vi "frog analysis.vi"(3 "error in (no error)":errorcluster, 5 "FROG in":refnum<class "FROG.lvclass">) -> (0 "error out":errorcluster, 2 "FROG out":refnum<class "FROG.lvclass">)   [LabVIEW 2020, in "FROG.lvclass"]
uses:
  FROG.lvclass
  FROG.lvclass/FROG.ctl
  Point Grey Camera/GUIcompressionCluster.ctl
  shared/OnOffTypeDef.ctl
  shared/CompressAndUpdate(Poly)/CompressAndUpdate(NumericArray).vi
  shared/CompressAndUpdate(Poly)/CompressAndUpdate(IMAQ Image).vi
  shared/CompressAndUpdate(Poly)/CompressAndUpdate(Numeric).vi
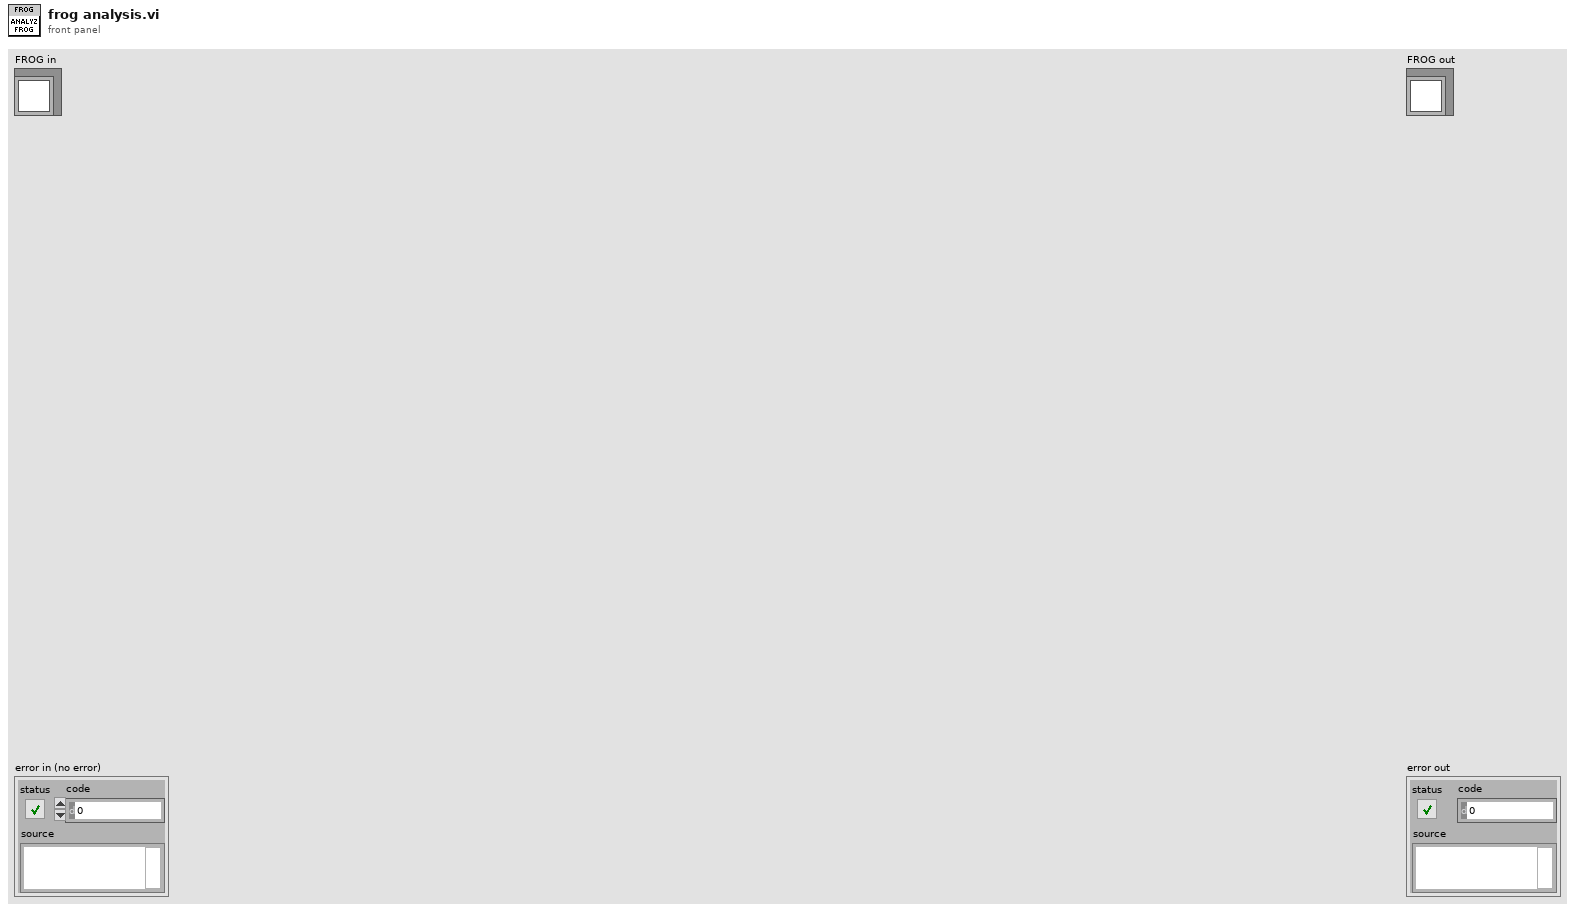
[diagram p1: front panel]
types:
  T1 = typedef "IMAQ Image.ctl" = refnum<image>
  T2 = typedef "GUIcompressionCluster.ctl" = cluster{"GUI8bit":T3, "GUICompression":T3, "CompressionQuality":i32}
  T3 = typedef "OnOffTypeDef.ctl" = enum16{"off", "on"}
  T4 = cluster{"waveout":dbl[], "specOut":dbl[], dbl[], "timeout":dbl[], "field":dbl[], dbl[]}
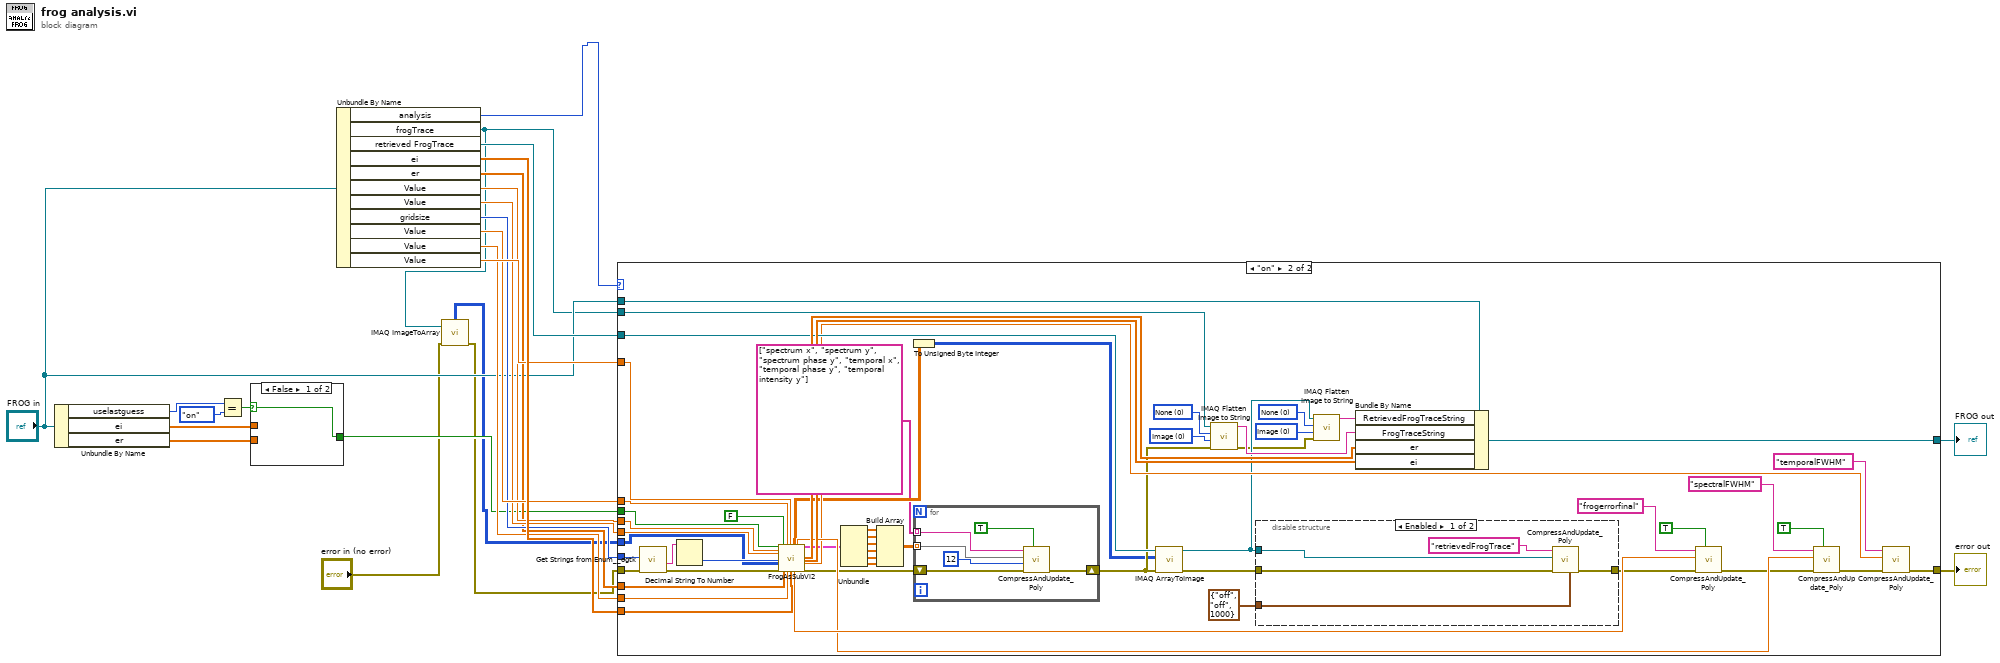
[diagram p0: block diagram]
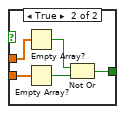
[diagram p2: hidden frame]
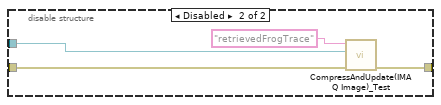
[diagram p4: hidden frame]
diagram:
  n1 = Unbundle By Name ("pressure read")("FROG in") -> ("uselastguess"=w10:enum16{"off", "on"}, "ei"=w9:dbl[], "er"=w8:dbl[])
  n2 = Equal?(x=w10, y=enum16{"off", "on"}."on" ("uselastguess")) -> (x = y?=w11:bool)
  n3 = case shown="False" w11 {
    selector: w11 -> [w24 _]
    tunnel: w9 -> [_ w25]
    tunnel: w8 -> [_ w29]
    tunnel: [w24 w26] -> w7
    frame False {
    }
    frame True {
      n4 = Empty Array?(array=w25) -> (empty?=w27:bool)
      n5 = Empty Array?(array=w29) -> (empty?=w28:bool)
      n6 = Not Or(1:w28, 2:w27) -> (0:w26:bool)
    }
  }
  n7 = Unbundle By Name ("pressure read")("FROG in") -> ("analysis"=w5:enum16{"off", "on"}, "frogTrace"=w4:T1, "retrieved FrogTrace"=w14:T1, "ei"=w21:dbl[], "er"=w13:dbl[], "Value"=w15:dbl, "Value"=w16:dbl, "gridsize"=w17:enum16{"64", "128", "256", "512"}, "Value"=w19:dbl, "Value"=w18:dbl, "Value"=w20:dbl)
  n8 = call "IMAQ ImageToArray"("error in (no error)"="error in (no error)", "Image"=w4) -> ("error out"=w1:errorcluster, "Image Pixels (U8)"=w3:u8[][])  [unwired: 2 in, 3 out]
  n9 = case shown="\"on\"" w5 {
    tunnel: "FROG in" -> [w31 w87]
    tunnel: [w31 w86] -> w22
    tunnel: w7 -> [_ w85]
    tunnel: w15 -> [_ w84]
    tunnel: w16 -> [_ w83]
    tunnel: w17 -> [_ w80]
    tunnel: w13 -> [_ w76]
    tunnel: w21 -> [_ w75]
    tunnel: w14 -> [_ w73]
    tunnel: [w30 w61] -> w23
    tunnel: w1 -> [w30 w51]
    tunnel: w19 -> [_ w49]
    tunnel: w20 -> [_ w48]
    tunnel: w18 -> [_ w47]
    tunnel: w4 -> [_ w42]
    tunnel: w3 -> [_ w34]
    frame "off", Default {
    }
    frame "on" {
      w39 = 0 items=["Image", "Image and Vision Info", "Reference to Image"] ("Type of Flatten (Image and Vision Info)")
      w38 = 0 items=["None", "JPEG", "PACKED BINARY"] ("Compression (None)")
      w43 = 0 items=["Image", "Image and Vision Info", "Reference to Image"] ("Type of Flatten (Image and Vision Info)")
      w44 = 0 items=["None", "JPEG", "PACKED BINARY"] ("Compression (None)")
      n10 = call <userlib>:"Get Strings from Enum__ogtk.vi"("error in (no error)"=w51, "Enum"=w80) -> ("error out"=w77:errorcluster, "String Value"=w79:string)  [unwired: 6 in, 2 out]
      n11 = Decimal String To Number(string=w79) -> (number=w78:i32)  [unwired: 2 in, 1 out]
      n12 = call "FrogAsSubVi2.vi"("use last retrieval as guess"=w85, "max time/retrieval [ms]"=w84, "set Frog error"=w83, "Grid size"=w78, "8-bit pixmap"=w34, "error in (no error)"=w77, "Stop"=FALSE, "er in"=w76, "delt"=w49, "dellam"=w47, "lam0"=w48, "ei in"=w75) -> ("retrieved Frog trace"=w60:dbl[][], "Best Frog Error"=w70:dbl, "spectral FWHM"=w67:dbl, "Temporal and Spatial Arrays"=w50:T4, "er"=w82:dbl[], "ei"=w81:dbl[], "temporal FWHM"=w65:dbl, "error out"=w46:errorcluster)  [unwired: 8 in]
      n13 = Unbundle(w50) -> ("waveout"=w59:dbl[], "specOut"=w58:dbl[], w57:dbl[], "timeout"=w56:dbl[], "field"=w55:dbl[], w54:dbl[])
      n14 = Build Array(w59, w58, w57, w56, w55, w54) -> (w53:dbl[][])
      n15 = To Unsigned Byte Integer(number=w60) -> (unsigned 8bit integer=w33:u8[][])
      n16 = for {
        tunnel: w53 -> [w101] mode=indexing
        tunnel: string[] ["spectrum x", "spectrum y", "spectrum phase y", "temporal x", "temporal phase y", "temporal intensity y"] -> [w102] mode=indexing
        shift-right: [w97] -> w41
        shift-left: w46 -> [w98]
        n17 = call-poly "CompressAndUpdate_Poly.vi"("force CVT update (false)"=TRUE, "error in"=w98, "precision (6)"=i16 12, "Numeric Array"=w101, "command or variable name"=w102) -> ("error out"=w97:errorcluster)  [unwired: 6 in]
      }
      n18 = call "IMAQ ArrayToImage"("error in (no error)"=w41, "Image Pixels (U8)"=w33, "Image"=w73) -> ("error out"=w64:errorcluster, "Image Out"=w37:T1)  [unwired: 7 in]
      n19 = call "IMAQ Flatten Image to String"("error in (no error)"=w41, "Type of Flatten (Image and Vision Info)"=w43, "Compression (None)"=w44, "Image"=w42) -> ("error out"=w36:errorcluster, "Data String"=w40:string)  [unwired: 6 in]
      n20 = disable-structure shown="Enabled" {
        disable-tunnel: w64 -> [w91 w96]
        disable-tunnel: [w90 w95] -> w45
        disable-tunnel: w37 -> [w89 w94]
        disable-tunnel: T2 {"GUI8bit"=enum."off", "GUICompression"=enum."off", "CompressionQuality"=1000} ("GUICompression") -> [w88 _]
        frame Enabled {
          n21 = call-poly "CompressAndUpdate_Poly.vi"("GUICompression"=w88, "error in"=w91, "IMAQ Image"=w89, "command or variable name"="retrievedFrogTrace") -> ("error out"=w90:errorcluster)  [unwired: 7 in]
        }
        frame Disabled {
          n22 = call "CompressAndUpdate(IMAQ Image)_Test.vi"("error in"=w96, "IMAQ Image"=w94, "command or variable name"="retrievedFrogTrace") -> ("error out"=w95:errorcluster)  [unwired: 8 in]
        }
      }
      n23 = call "IMAQ Flatten Image to String"("error in (no error)"=w36, "Type of Flatten (Image and Vision Info)"=w39, "Compression (None)"=w38, "Image"=w37) -> ("Data String"=w35:string)  [unwired: 6 in, 1 out]
      n24 = Bundle By Name(cluster=w87, "RetrievedFrogTraceString"=w35, "FrogTraceString"=w40, "er"=w82, "ei"=w81) -> (w86:refnum<class "FROG.lvclass">)
      n25 = call-poly "CompressAndUpdate_Poly.vi"("force CVT update (false)"=TRUE, "error in"=w45, "Numeric"=w70, "command or variable name"="frogerrorfinal") -> ("error out"=w63:errorcluster)  [unwired: 7 in]
      n26 = call-poly "CompressAndUpdate_Poly.vi"("force CVT update (false)"=TRUE, "error in"=w63, "Numeric"=w67, "command or variable name"="spectralFWHM") -> ("error out"=w62:errorcluster)  [unwired: 7 in]
      n27 = call-poly "CompressAndUpdate_Poly.vi"("error in"=w62, "Numeric"=w65, "command or variable name"="temporalFWHM") -> ("error out"=w61:errorcluster)  [unwired: 8 in]
    }
  }
  "error out" <- w23
  "FROG out" <- w22
